vi "Check Averaging.vi"(6 "Timeout [s]":dbl=10.0, 8 "Error In":errorcluster, 10 "Averaging":T1 {"Traces" min=1 max=200 step=1}, 11 "Result Queue":refnum<queue>) -> (0 "Error Out":errorcluster, 2 "Ready":bool)   [LabVIEW 2019]
uses:
  Controls/Acquisition Result.ctl
  Averaging.ctl
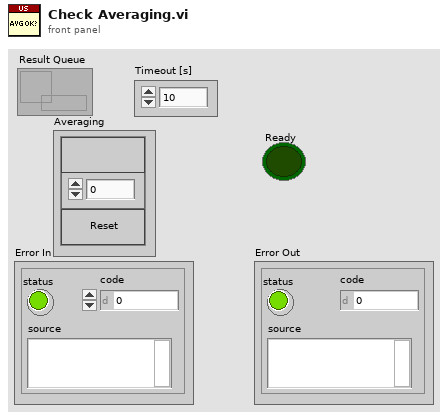
[diagram p1: front panel]
types:
  T1 = typedef "Averaging.ctl" = cluster{"On":bool, "Traces":i32, "Reset":bool}
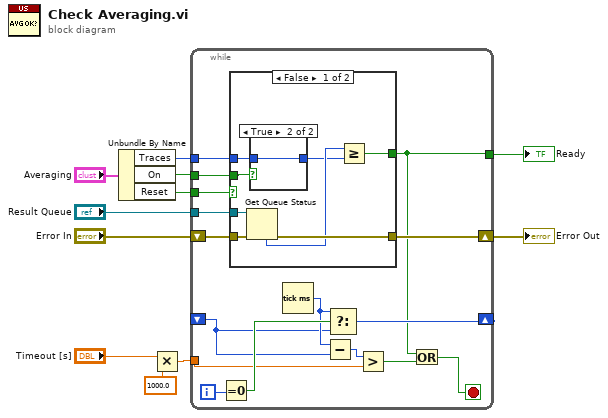
[diagram p0: block diagram]
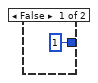
[diagram p2: hidden frame]
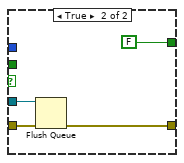
[diagram p3: hidden frame]
diagram:
  n1 = Unbundle By Name("Averaging") -> ("Traces"=w10:i32, "On"=w9:bool, "Reset"=w8:bool)
  n2 = Multiply(x="Timeout [s]", y=1000.0) -> (x*y=w1:dbl)
  n3 = while {
    tunnel: w10 -> [w26]
    tunnel: w8 -> [w24]
    tunnel: "Result Queue" -> [w23]
    shift-right: [w27] -> w11
    shift-left: "Error In" -> [w22]
    tunnel: w9 -> [w25]
    tunnel: [w15] -> w4
    shift-right: [w20] -> _
    shift-left: _ -> [w12]
    tunnel: w1 -> [w17]
    i -> [w14]
    stop <- w13 stop-if-true
    n4 = Equal To 0?(x=w14) -> (x = 0?=w21:bool)
    n5 = case shown="False" w24 {
      tunnel: [w35 w40] -> w27
      tunnel: w23 -> [w34 w39]
      tunnel: w26 -> [w30 _]
      tunnel: [w28 FALSE] -> w15
      tunnel: w25 -> [w31 _]
      tunnel: w22 -> [w32 w41]
      frame False {
        n6 = Get Queue Status(queue=w34, error in (no error)=w32) -> (error out=w35:errorcluster, # elements in queue=w33:i32)  [unwired: 1 in, 6 out]
        n7 = case shown="True" w31 {
          tunnel: [1 ("f") w37] -> w29
          tunnel: w30 -> [_ w37]
          frame False {
          }
          frame True {
          }
        }
        n8 = Greater Or Equal?(x=w33, y=w29) -> (x >= y?=w28:bool)
      }
      frame True {
        n9 = Flush Queue(queue=w39, error in (no error)=w41) -> (error out=w40:errorcluster)  [unwired: 2 out]
      }
    }
    n10 = Tick Count (ms)() -> (millisecond timer value=w19:u32)
    n11 = Subtract(x=w19, y=w12) -> (x-y=w18:u32)
    n12 = Select(t=w19, s=w21, f=w12) -> (s? t:f=w20:u32)
    n13 = Greater?(x=w18, y=w17) -> (0:w16:bool)
    n14 = Or(x=w15, y=w16) -> (x .or. y?=w13:bool)
  }
  "Error Out" <- w11
  "Ready" <- w4
